vi "Delete_Commands.vi"(1 "Command Indices":i32[](array[numeric]), 2 "Input Sequence":cluster{string, string[], dbl[], dbl}[](array[cluster])) -> (0 "Output Sequence":cluster{string, string[], dbl[], dbl}[](array[cluster]))   [LabVIEW 2011]
doc: "Deletes the commands at the given indices from the sequence. Additionally, this VI will delete all commands with an API_ID matching the API_ID of any commands at the given indices."
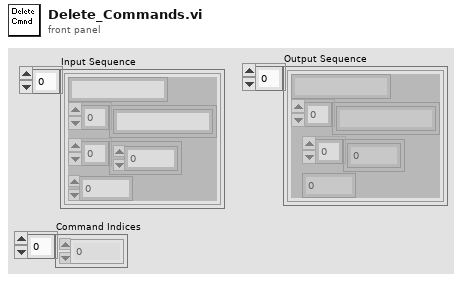
[diagram p1: front panel]
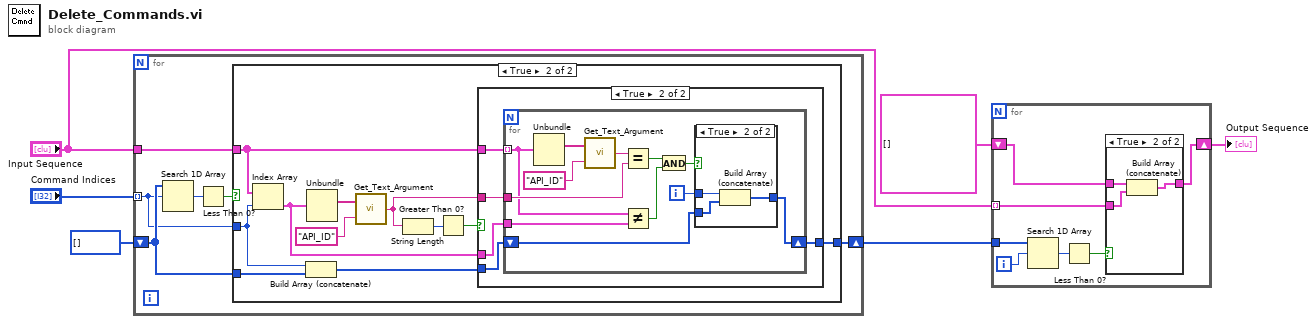
[diagram p0: block diagram]
diagram:
  n1 = for {
    tunnel: "Input Sequence" -> [w12]
    tunnel: "Command Indices" -> [w9] mode=indexing
    shift-right: [w11] -> w3
    shift-left: i32[] [] -> [w10]
    n2 = Search 1D Array(1D array=w10, element=w9) -> (index of element=w8:i32)  [unwired: 1 in]
    n3 = Less Than 0?(x=w8) -> (x < 0?=w7:bool)
    n4 = case shown="True" w7 {
      tunnel: w12 -> [_ w14]
      tunnel: [w13 w19] -> w11
      tunnel: w10 -> [w13 w18]
      tunnel: w9 -> [_ w16]
      frame False {
      }
      frame True {
        n5 = Index Array(array=w14, index=w16) -> (element=w15:cluster{string, string[], dbl[], dbl})
        n6 = Build Array (concatenate)(w16, w18) -> (w17:i32[])
        n7 = Unbundle(w15) -> (w24:string[])  [unwired: 3 out]
        n8 = call "Get_Text_Argument.vi"("Argument"="API_ID", "Argument List"=w24) -> ("Text"=w22:string)
        n9 = String Length(string=w22) -> (length=w21:i32)
        n10 = Greater Than 0?(x=w21) -> (x > 0?=w20:bool)
        n11 = case shown="True" w20 {
          tunnel: w14 -> [_ w30]
          tunnel: w22 -> [_ w29]
          tunnel: w15 -> [_ w28]
          tunnel: [w25 w27] -> w19
          tunnel: w17 -> [w25 w26]
          frame False {
          }
          frame True {
            n12 = for {
              tunnel: w30 -> [w38] mode=indexing
              tunnel: w29 -> [w39]
              tunnel: w28 -> [w37]
              shift-right: [w32] -> w27
              shift-left: w26 -> [w31]
              i -> [w33]
              n13 = Unbundle(w38) -> (w41:string[])  [unwired: 3 out]
              n14 = call "Get_Text_Argument.vi"("Argument"="API_ID", "Argument List"=w41) -> ("Text"=w40:string)
              n15 = Equal?(x=w40, y=w39) -> (x = y?=w36:bool)
              n16 = Not Equal?(x=w38, y=w37) -> (x != y?=w35:bool)
              n17 = And(x=w36, y=w35) -> (x .and. y?=w34:bool)
              n18 = case shown="True" w34 {
                tunnel: w33 -> [_ w45]
                tunnel: [w43 w46] -> w32
                tunnel: w31 -> [w43 w44]
                frame False {
                }
                frame True {
                  n19 = Build Array (concatenate)(w45, w44) -> (w46:i32[])
                }
              }
            }
          }
        }
      }
    }
  }
  n20 = for {
    tunnel: "Input Sequence" -> [w48] mode=indexing
    tunnel: w3 -> [w52]
    shift-right: [w47] -> w1
    shift-left: cluster{string, string[], dbl[], dbl}[] [] ("Input Sequence") -> [w49]
    i -> [w53]
    n21 = Search 1D Array(1D array=w52, element=w53) -> (index of element=w51:i32)  [unwired: 1 in]
    n22 = Less Than 0?(x=w51) -> (x < 0?=w50:bool)
    n23 = case shown="True" w50 {
      tunnel: w49 -> [w54 w56]
      tunnel: w48 -> [_ w57]
      tunnel: [w54 w55] -> w47
      frame False {
      }
      frame True {
        n24 = Build Array (concatenate)(w56, w57) -> (w55:cluster{string, string[], dbl[], dbl}[])
      }
    }
  }
  "Output Sequence" <- w1
